vi "Create PUBLISH Packet (Server).vi"(4 "RETAIN":bool, 5 "PUBLISH type":refnum<class "PUBLISH.lvclass">, 6 "QoS":T1, 7 "DUP (Re-delivery attempt)":bool, 8 "error in (no error)":errorcluster, 9 "Packet ID (empty: generate new)":u16 format="%04x", 10 "Payload":u8[](array[numeric]) format="%08b", 11 "Topic Name":string) -> (0 "error out":errorcluster, 1 "Packet ID":u16 format="%04x", 3 "PUBLISH":refnum<class "PUBLISH.lvclass">)   [LabVIEW 2013, in "PUBLISH.lvclass"]
uses:
  PUBLISH.lvclass
  ControlPacket/QualityOfService -- enum.ctl
  PUBLISH.lvclass/PUBLISH.ctl
  ControlPacket/ControlPacket.lvclass/ControlPacket.ctl
  ControlPacket/ControlPacket.lvclass
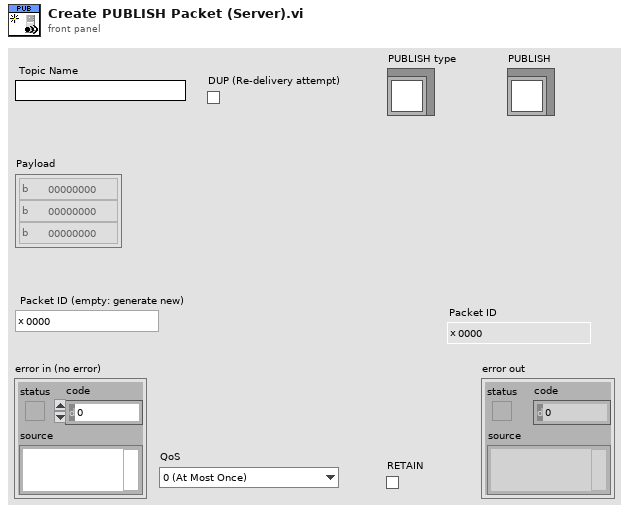
[diagram p1: front panel]
types:
  T1 = typedef "ControlPacket.lvclass/QualityOfService -- enum.ctl" = enum16{"0 (At Most Once)", "1 (At Least Once)", "2 (Exactly Once)"}
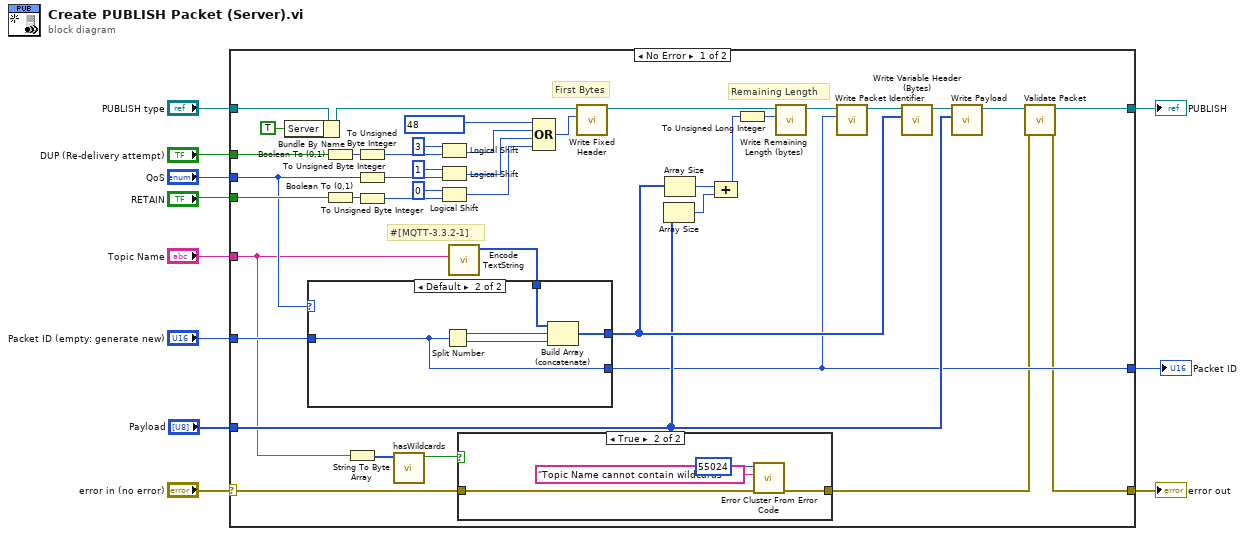
[diagram p0: block diagram]
diagram:
  n1 = case shown="No Error" "error in (no error)" {
    selector: "error in (no error)" -> [w13 w64]
    tunnel: [w21 w64] -> w10
    tunnel: [w22 w63] -> w8
    tunnel: "PUBLISH type" -> [w18 w63]
    tunnel: "DUP (Re-delivery attempt)" -> [w38 _]
    tunnel: "RETAIN" -> [w51 _]
    tunnel: "QoS" -> [w20 _]
    tunnel: "Topic Name" -> [w15 _]
    tunnel: "Packet ID (empty: generate new)" -> [w25 _]
    tunnel: "Payload" -> [w31 _]
    tunnel: [w24 _] -> w1
    frame No Error {
      # "#[MQTT-3.3.2-1]"
      # "Remaining Length"
      # "First Bytes"
      n2 = Bundle By Name(cluster=w18, "Server"=TRUE) -> (w17:refnum<class "PUBLISH.lvclass">)
      n3 = Boolean To (0,1)(Boolean=w38) -> (0, 1=w47:i16)
      n4 = Boolean To (0,1)(Boolean=w51) -> (0, 1=w46:i16)
      n5 = String To Byte Array(string=w15) -> (unsigned byte array=w16:u8[])
      n6 = To Unsigned Byte Integer(number=w47) -> (unsigned 8bit integer=w48:u8)
      n7 = To Unsigned Byte Integer(number=w20) -> (unsigned 8bit integer=w45:u8)
      n8 = To Unsigned Byte Integer(number=w46) -> (unsigned 8bit integer=w44:u8)
      n9 = call "hasWildcards.vi"("Topic Name (Bytes Array)"=w16) -> ("has Wildcards"=w14:bool)  [unwired: 10 in]
      n10 = Logical Shift(y=i16 3, x=w48) -> (x << y=w49:u8)
      n11 = Logical Shift(y=i16 1, x=w45) -> (x << y=w43:u8)
      n12 = Logical Shift(y=i16 0, x=w44) -> (x << y=w42:u8)
      n13 = call "Encode TextString.vi"("Text String"=w15) -> ("Length-Prefixed Field"=w33:u8[])  [unwired: 10 in]
      n14 = case shown="Default" w20 {
        tunnel: w33 -> [w57 w62]
        tunnel: [w57 w59] -> w32
        tunnel: w25 -> [_ w58]
        tunnel: [_ w58] -> w24
        frame "0 (At Most Once)" {
          # "#[MQTT-2.3.1-5]"
        }
        frame Default {
          n15 = Split Number(x=w58) -> (hi(x)=w61:u8, lo(x)=w60:u8)
          n16 = Build Array (concatenate)(w62, w61, w60) -> (w59:u8[])
        }
      }
      n17 = case shown="True" w14 {
        tunnel: w13 -> [w52 w55]
        tunnel: [w52 w56] -> w12
        frame False {
        }
        frame True {
          n18 = call <vilib>:"Error Cluster From Error Code.vi"("error in (no error)"=w55, "error message (\"\")"="Topic Name cannot contain wildcards" ("error message (\"\")"), "error code (0)"=55024) -> ("error out"=w56:errorcluster)  [unwired: 6 in]
        }
      }
      n19 = Compound Arithmetic op=OR(u8 48, w49, w43, w42) -> (w37:u8)
      n20 = call "Write Fixed Header.vi"("Fixed Header"=w37, "ControlPacket in"=w17) -> ("ControlPacket out"=w35:refnum<class "PUBLISH.lvclass">)  [unwired: 9 in]
      n21 = Array Size(array=w31) -> (size(s)=w29:i32)
      n22 = Array Size(array=w32) -> (size(s)=w30:i32)
      n23 = Compound Arithmetic op=ADD(w30, w29) -> (w28:i32)
      n24 = To Unsigned Long Integer(number=w28) -> (unsigned 32bit integer=w36:u32)
      n25 = call "Write Remaining Length (bytes).vi"("Remaining Length (bytes)"=w36, "ControlPacket in"=w35) -> ("ControlPacket out"=w27:refnum<class "PUBLISH.lvclass">)  [unwired: 9 in]
      n26 = call "Write Packet Identifier.vi"("Packet Identifier"=w24, "ControlPacket in"=w27) -> ("ControlPacket out"=w26:refnum<class "PUBLISH.lvclass">)  [unwired: 9 in]
      n27 = call "Write Variable Header (Bytes).vi"("Variable Header (Bytes)"=w32, "ControlPacket in"=w26) -> ("ControlPacket out"=w34:refnum<class "PUBLISH.lvclass">)  [unwired: 9 in]
      n28 = call "Write Payload.vi"("Payload"=w31, "ControlPacket in"=w34) -> ("ControlPacket out"=w23:refnum<class "PUBLISH.lvclass">)  [unwired: 9 in]
      n29 = call "Validate Packet.vi"("error in (no error)"=w12, "ControlPacket in"=w23) -> ("error out"=w21:errorcluster, "ControlPacket out"=w22:refnum<class "PUBLISH.lvclass">)  [unwired: 8 in]
    }
    frame Error {
    }
  }
  "error out" <- w10
  "PUBLISH" <- w8
  "Packet ID" <- w1
